vi "Decode Points Referee.vi"(7 "Boolean":bool=TRUE, 8 "error in":errorcluster, 9 "array":u8[](array[numeric]), 10 "Key":i32=5) -> (0 "error out":errorcluster, 1 "array w/ subset deleted out":u8[](array[numeric]), 3 "Point":cluster{"x":sgl, "y":sgl})   [LabVIEW 2016]
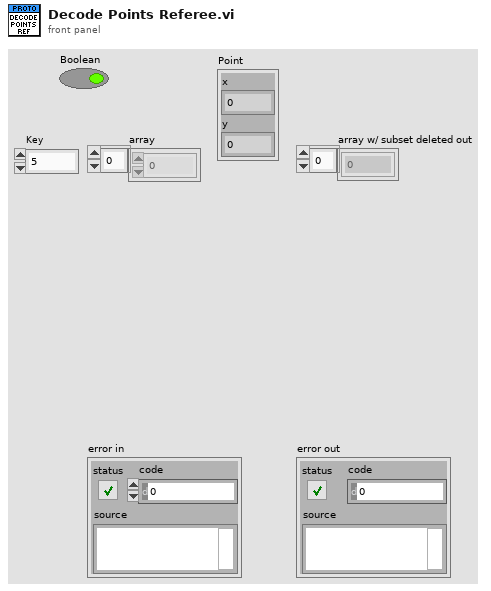
[diagram p1: front panel]
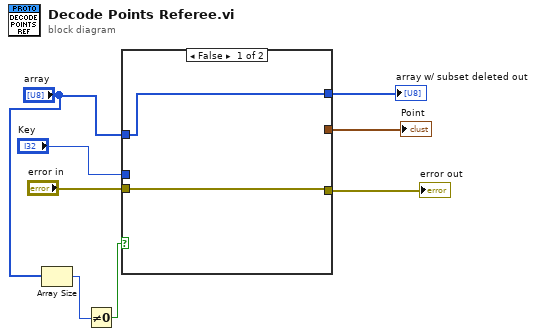
[diagram p0: block diagram]
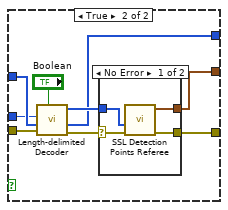
[diagram p2: hidden frame]
diagram:
  n1 = Array Size(array="array") -> (size(s)=w3:i32)
  n2 = Not Equal To 0?(x=w3) -> (x != 0?=w2:bool)
  n3 = case shown="False" w2 {
    tunnel: "array" -> [w10 w16]
    tunnel: "Key" -> [_ w15]
    tunnel: "error in" -> [w9 w14]
    tunnel: [w10 w13] -> w6
    tunnel: [w9 w12] -> w5
    tunnel: [_ w11] -> w4
    frame False {
    }
    frame True {
      n4 = call "Length-delimited Decoder.vi"("Optional"="Boolean", "error in (no error)"=w14, "Array"=w16, "Key"=w15) -> ("error out"=w18:errorcluster, "array w/ subset deleted"=w13:u8[], "Length-delimited"=w17:u8[])  [unwired: 4 in, 1 out]
      n5 = case shown="No Error" w18 {
        selector: w18 -> [w22 w24]
        tunnel: [w23 w24] -> w12
        tunnel: w17 -> [w21 _]
        tunnel: [w20 _] -> w11
        frame No Error {
          n6 = call "SSL Detection Points Referee.vi"("error in"=w22, "Array"=w21) -> ("error out"=w23:errorcluster, "Point"=w20:cluster{"x":sgl, "y":sgl})  [unwired: 7 in, 1 out]
        }
        frame Error {
        }
      }
    }
  }
  "error out" <- w5
  "array w/ subset deleted out" <- w6
  "Point" <- w4
